vi "Image Request.vi"(8 "error in (no error)":errorcluster, 11 "Controller in":refnum<class "Controller.lvclass">) -> (0 "error out":errorcluster, 3 "Controller out":refnum<class "Controller.lvclass">)   [LabVIEW 2022 SP3, in "Controller.lvlib" / "Controller.lvclass"]
uses:
  Controller.lvclass
  Controller.lvclass/Controller.ctl
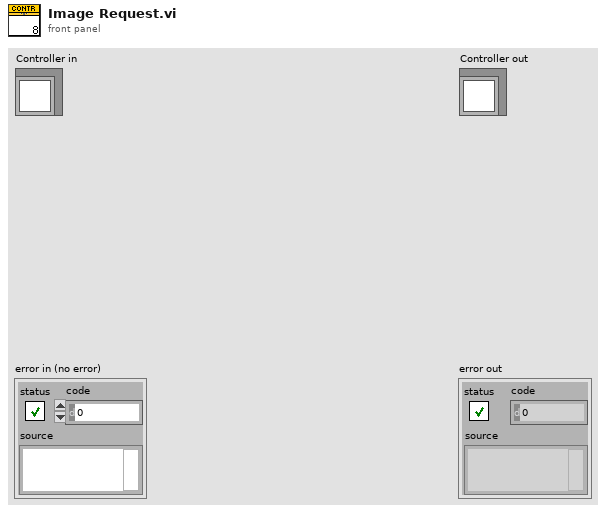
[diagram p1: front panel]
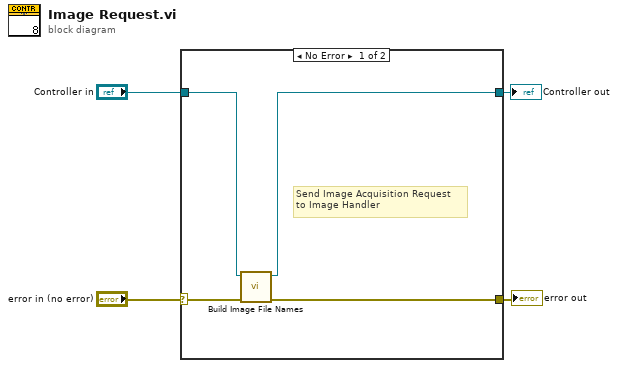
[diagram p0: block diagram]
diagram:
  n1 = case shown="No Error" "error in (no error)" {
    selector: "error in (no error)" -> [w8 w9]
    tunnel: "Controller in" -> [w6 w10]
    tunnel: [w5 w10] -> w2
    tunnel: [w7 w9] -> w1
    frame No Error {
      # "Send Image Acquisition Request\nto Image Handler"
      n2 = call "Build Image File Names.vi"("error in (no error)"=w8, "Controller in"=w6) -> ("error out"=w7:errorcluster, "Controller out"=w5:refnum<class "Controller.lvclass">)  [unwired: 7 in, 1 out]
    }
    frame Error {
    }
  }
  "error out" <- w1
  "Controller out" <- w2
